vi "BeadCoolerFixedZ(SubVI)_noint.vi"(1 "AI0":i16, 2 "Dc Pos":i16, 6 "lp coeff":i32[](array[numeric])=[-955995012, 2025731616, 1001305, -1023351008, 2092954700, 1034533], 7 "dg":fxp<+/-,24,12>, 8 "hp coeff":i32[](array[numeric])=[946630756, 1010186290], 13 "Upper lim":fxp<+/-,16,16>, 14 "Lower lim":fxp<+/-,16,16>) -> (10 "Output":fxp<+/-,16,16>)   [LabVIEW 2013]
uses:
  <vilib>/rvi/FXPMathLib/FxpInterpret/XNode/nifxpmath_Interpret.xnode
  <vilib>/rvi/Analysis/measure/butterworth/XNode/niFpgaButterworthFilter.xnode
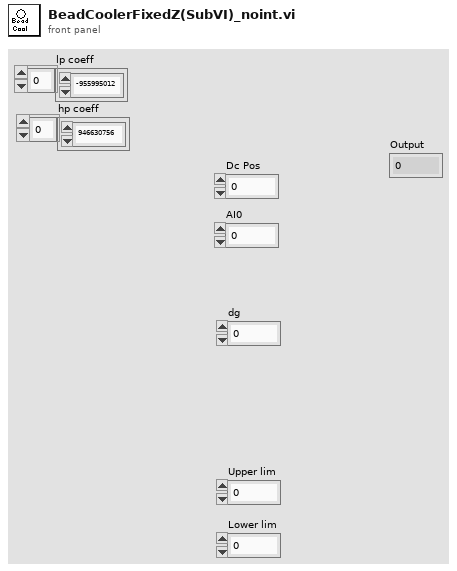
[diagram p1: front panel]
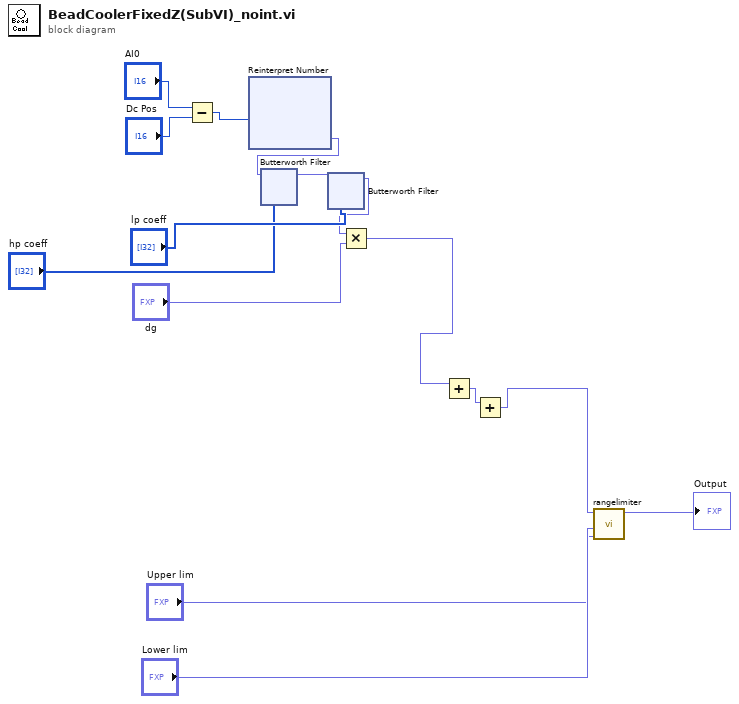
[diagram p0: block diagram]
diagram:
  n1 = Subtract(x="AI0", y="Dc Pos") -> (x-y=w11:i16)
  n2 = xnode "Reinterpret Number"("x"=w11) -> ("y"=w1:fxp<+/-,16,16>)
  n3 = xnode "Butterworth Filter"("input data"=w1, "scaled coefficients"="hp coeff") -> ("output data"=w4:fxp<+/-,20,20>)  [unwired: 1 in]
  n4 = xnode "Butterworth Filter"("input data"=w4, "scaled coefficients"="lp coeff") -> ("output data"=w3:fxp<+/-,24,24>)  [unwired: 1 in]
  n5 = Multiply(x=w3, y="dg") -> (x*y=w2:fxp<+/-,24,23>)
  n6 = Add(x=w2) -> (y=w16:fxp<+/-,24,23>, x+y=w8:fxp<+/-,24,23>)
  n7 = Add(x=w8) -> (x+y=w7:fxp<+/-,16,16>)  [unwired: 1 in]
  n8 = call "rangelimiter.vi"("Upper lim"="Upper lim", "Lower lim"="Lower lim", "Input"=w7) -> ("Output"=→"Output":fxp<+/-,16,16>)  [unwired: 8 in]
